vi "流量计全局变量.vi"() -> ()   [LabVIEW 2016]
panel:
  in  "运行间隔":i16=4 min=1 max=24
  in  "数量 3":u16
  in  "数量 2":u16
  in  "数量":u16
  in  "流量计启用 3":bool
  in  "流量计启用 2":bool
  in  "流量计启用":bool
  out "总累积流量":dbl
  out "总流量":dbl
  out "平均流速":dbl
  out "平均水位":dbl
  out "TX Timestamp":timestamp
  out "TX Data":string
  out "RX Timestamp":timestamp
  out "RX Data":string
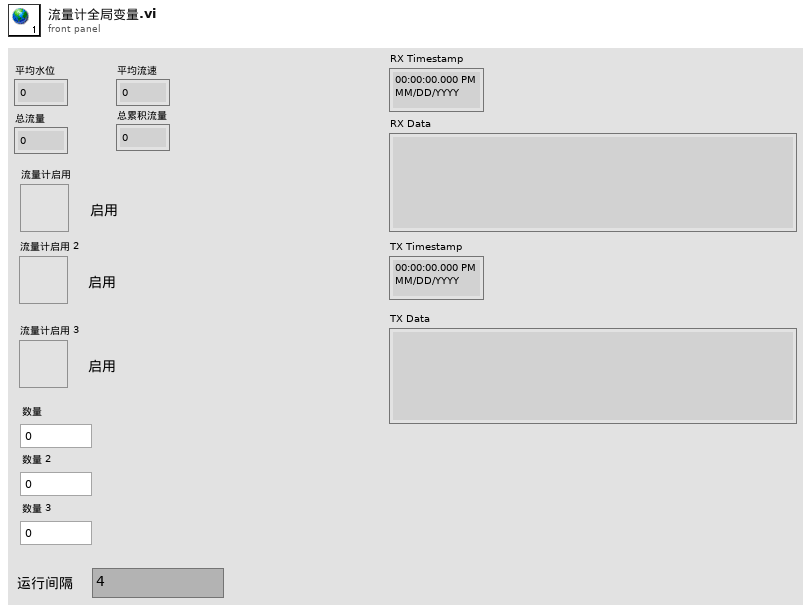
[diagram p1: front panel]
diagram:
